vi "fetch_and_translate_trigger.vi"(8 "error in (no error)":errorcluster, 11 "ImagingModeDL091001Scaffold in":refnum<class "ImagingModeDL091001Scaffold.lvclass">) -> (0 "error out":errorcluster, 1 "sender TLC type":T1=enum."ImagingMode", 2 "statechart trigger":T2, 3 "ImagingModeDL091001Scaffold out":refnum<class "ImagingModeDL091001Scaffold.lvclass">)   [LabVIEW 2010, in "ImagingModeDL091001Scaffold.lvclass"]
uses:
  ImagingModeDL091001Scaffold.lvclass
  internal_triggers_enum.ctl
  common/enumerations/top-level_component_type_enum.ctl
  GenericImagingMode/GenericImagingMode/trigger_enum.ctl
  GenericImagingMode/GenericImagingMode/GenericImagingMode.lvclass
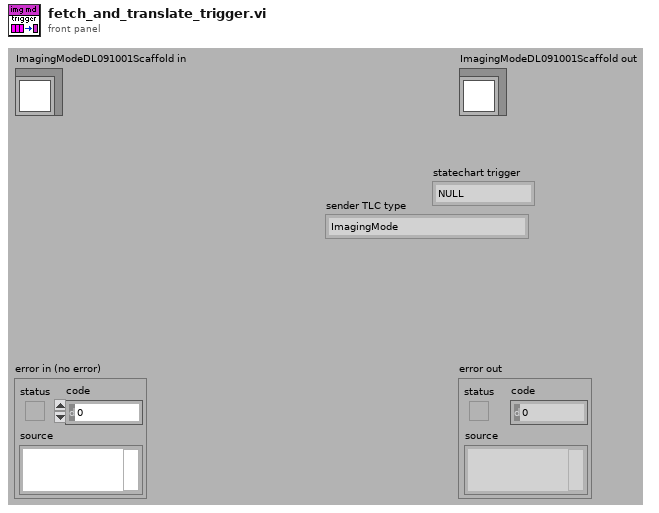
[diagram p1: front panel]
types:
  T1 = typedef "top-level_component_type_enum.ctl" = enum16{"undefined", "ImagingMode", "ScanHead", "DAQ", "ImageAssembler", "Display", "DataCollection", "Analyser", "Stimulator", "ExperimentController", "Instrument", "Stage"}
  T2 = typedef "ImagingModeDL091001Scaffold.lvclass/internal_triggers_enum.ctl" = enum16{"NULL", "initialise", "terminate", "start sweep", "stop sweep", "update", "proceed", "draw overlay", "attach observer", "detach observer", "finish sweep"}
  T3 = typedef "GenericImagingMode.lvclass/trigger_enum.ctl" = enum16{"NULL", "proceed"}
  T4 = typedef "GenericToplevelComponent.lvclass/common_trigger_enum.ctl" = enum16{"NULL", "initialise", "terminate", "fetch command", "fetch data", "attach observer", "register as observer", "detach observer", "acknowledge", "start", "stop", "sweep started", "sweep finished", "experiment started", "experiment stopped"}
  T5 = typedef "trigger_type_enum.ctl" = enum8{"external", "internal", "common"}
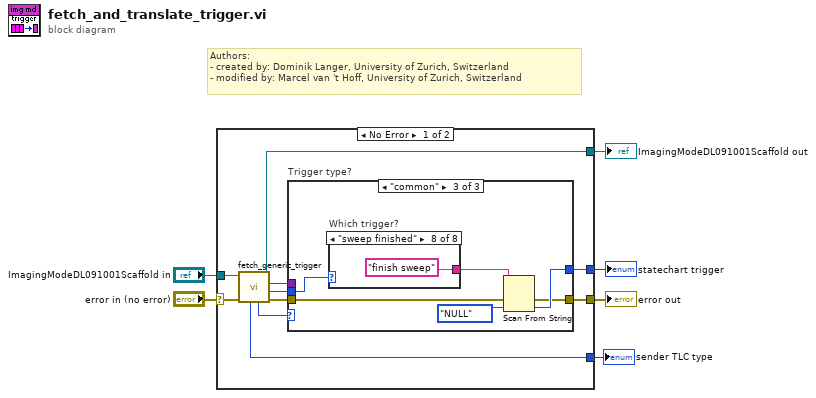
[diagram p0: block diagram]
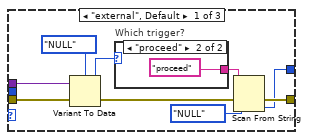
[diagram p2: hidden frame]
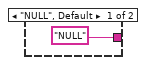
[diagram p3: hidden frame]
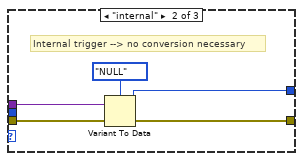
[diagram p4: hidden frame]
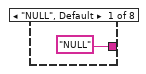
[diagram p5: hidden frame]
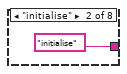
[diagram p6: hidden frame]
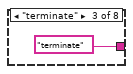
[diagram p7: hidden frame]
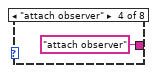
[diagram p8: hidden frame]
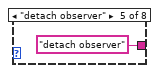
[diagram p9: hidden frame]
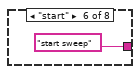
[diagram p10: hidden frame]
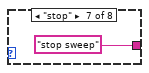
[diagram p11: hidden frame]
diagram:
  # "Authors: \n- created by: Dominik Langer, University of Zurich, Switzerland\n- modified by: Marcel van 't Hoff, University of Zurich, Switzerland"
  n1 = case shown="No Error" "error in (no error)" {
    selector: "error in (no error)" -> [w14 w48]
    tunnel: [w16 w48] -> w5
    tunnel: [w11 w47] -> w3
    tunnel: "ImagingModeDL091001Scaffold in" -> [w12 w47]
    tunnel: [w15 _] -> w2
    tunnel: [w7 _] -> w1
    frame No Error {
      n2 = call-dynamic "fetch_generic_trigger.vi"("error in (no error)"=w14, "GenericToplevelComponent in"=w12) -> ("error out"=w13:errorcluster, "common trigger"=w8:T4, "trigger"=w9:variant, "GenericToplevelComponent out"=w11:refnum<class "ImagingModeDL091001Scaffold.lvclass">, "trigger type"=w10:T5, "sender TLC type"=w7:T1)  [unwired: 3 in, 1 out]
      n3 = case "Trigger type?" shown="\"common\"" w10 {
        tunnel: [w19 w31 w33] -> w16
        tunnel: [w18 w29 w36] -> w15
        tunnel: w13 -> [w22 w32 w34]
        tunnel: w9 -> [w23 w30 _]
        tunnel: w8 -> [_ _ w38]
        frame "external", Default {
          n4 = Variant To Data(error in=w22, Variant=w23, type=trigger_enum."NULL" ("message")) -> (error out=w20:errorcluster, data=w25:T3)
          n5 = case "Which trigger?" shown="\"proceed\"" w25 {
            tunnel: ["NULL" "proceed"] -> w17
            frame "NULL", Default {
            }
            frame "proceed" {
            }
          }
          n6 = Scan From String(input string=w17, error in=w20, default 1=internal_triggers_enum."NULL" ("statechart trigger")) -> (error out=w19:errorcluster, output 1=w18:T2)  [unwired: 2 in, 2 out]
        }
        frame "internal" {
          # "Internal trigger --> no conversion necessary"
          n7 = Variant To Data(error in=w32, Variant=w30, type=internal_triggers_enum."NULL" ("statechart trigger")) -> (error out=w31:errorcluster, data=w29:T2)
        }
        frame "common" {
          n8 = case "Which trigger?" shown="\"sweep finished\"" w38 {
            tunnel: ["NULL" "initialise" "terminate" "attach observer" "detach observer" "start sweep" "stop sweep" "finish sweep"] -> w35
            frame "NULL", Default {
            }
            frame "initialise" {
            }
            frame "terminate" {
            }
            frame "attach observer" {
            }
            frame "detach observer" {
            }
            frame "start" {
            }
            frame "stop" {
            }
            frame "sweep finished" {
            }
          }
          n9 = Scan From String(input string=w35, error in=w34, default 1=internal_triggers_enum."NULL" ("statechart trigger")) -> (error out=w33:errorcluster, output 1=w36:T2)  [unwired: 2 in, 2 out]
        }
      }
    }
    frame Error {
    }
  }
  "error out" <- w5
  "ImagingModeDL091001Scaffold out" <- w3
  "statechart trigger" <- w2
  "sender TLC type" <- w1
